vi "sub_conv_map_gen_v2.vi"(11 "code type":T1(ring)) -> (1 "output in decimal":u32[][](array[numeric]), 3 "state transition":u32[][](array[numeric]))   [LabVIEW 2014]
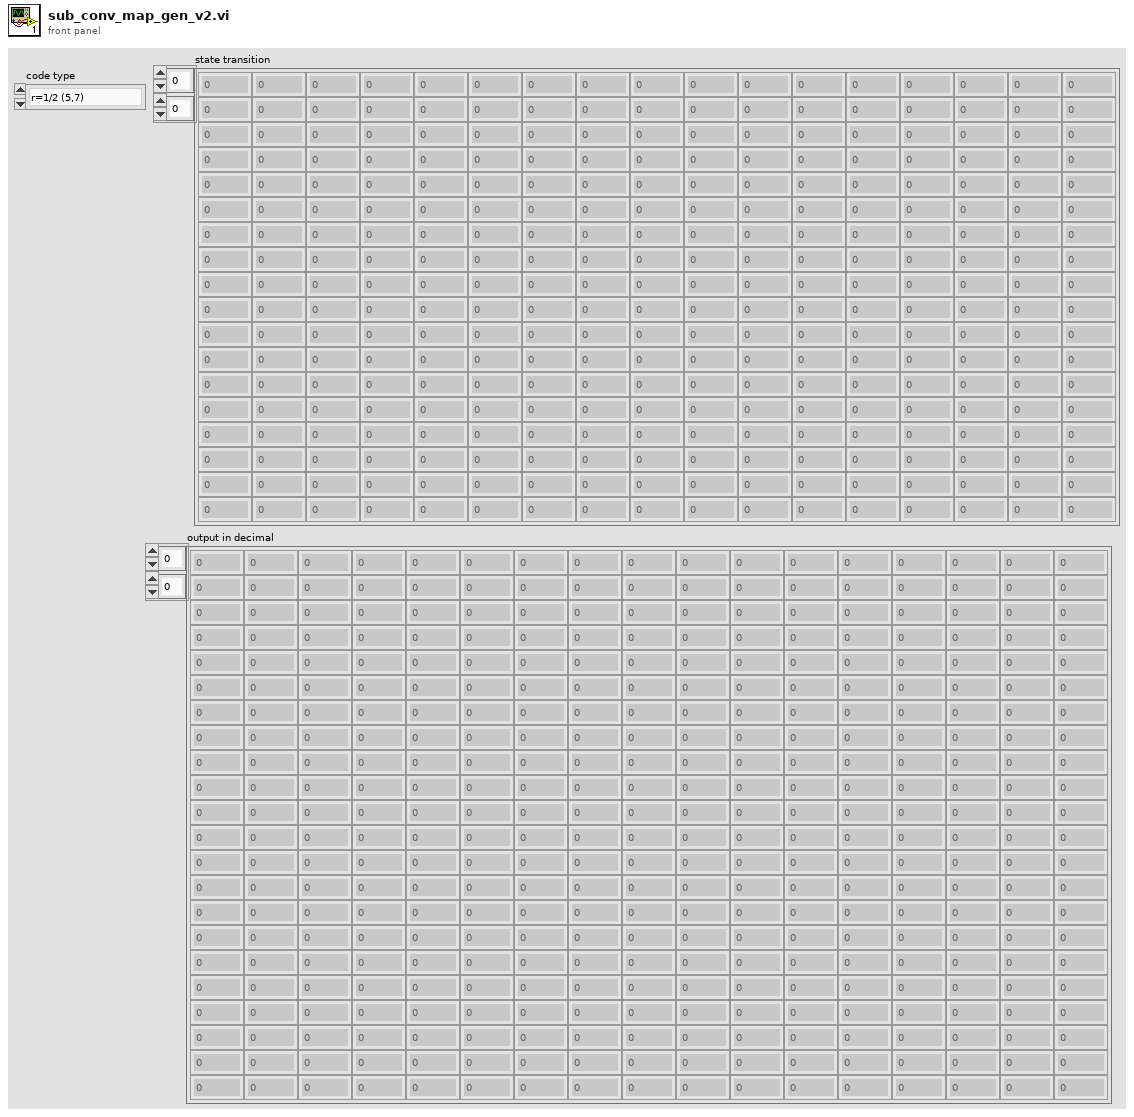
[diagram p1: front panel]
types:
  T1 = enum16{"r=1/2 (5,7)", "r=1/2 (13,17)", "r=1/4 (25,27,33,37)"}
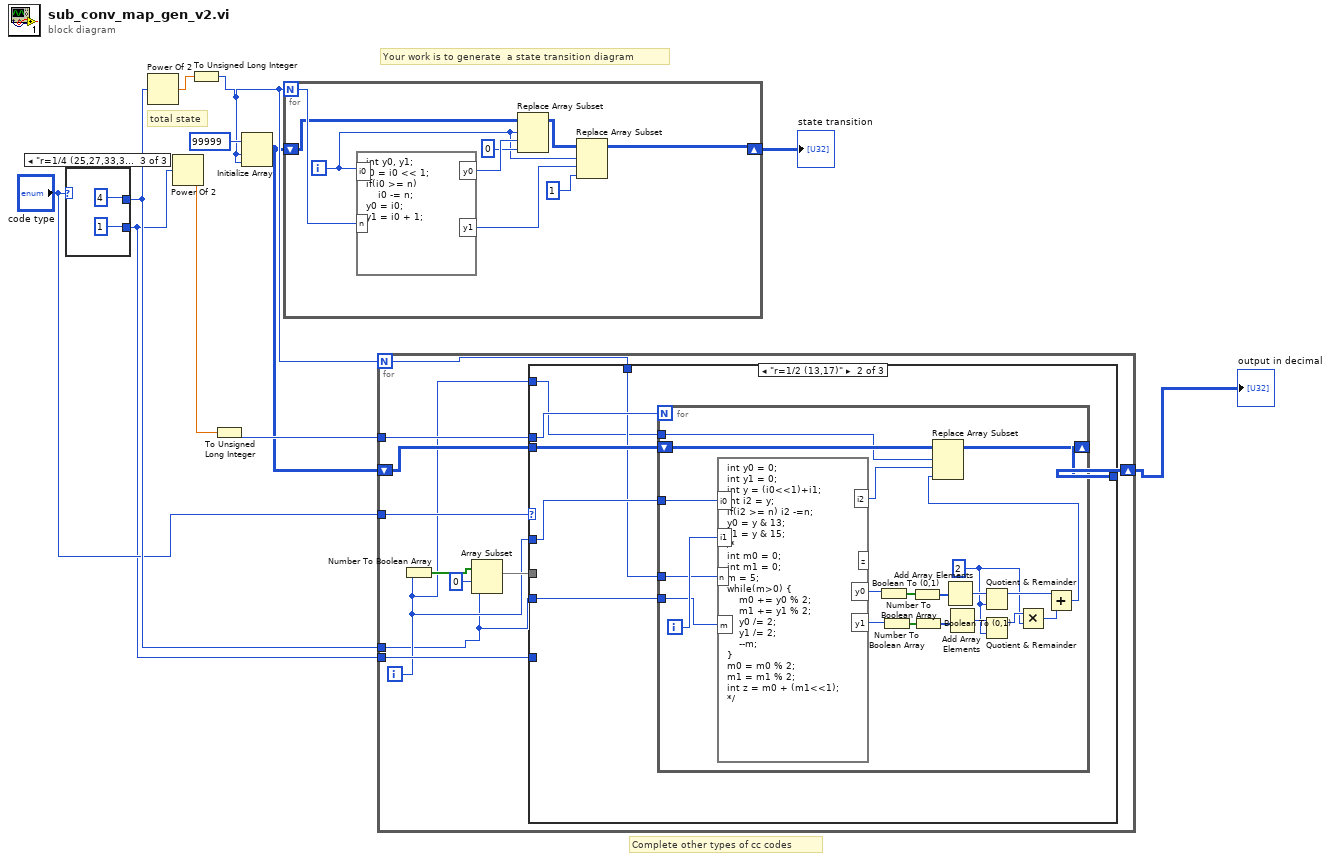
[diagram p0: block diagram]
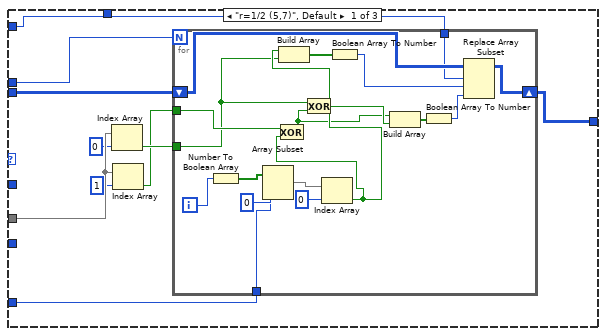
[diagram p2: hidden frame]
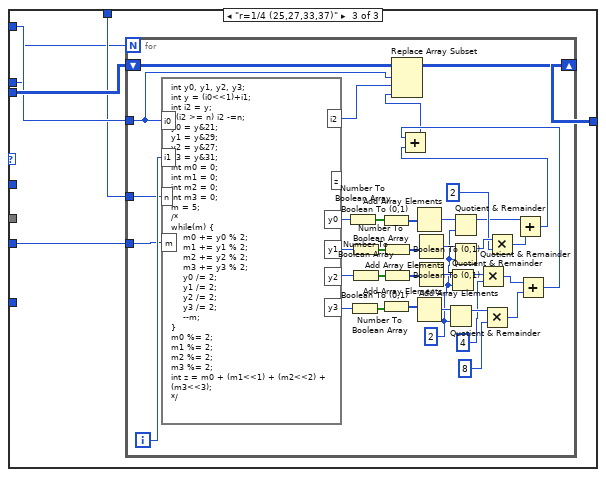
[diagram p3: hidden frame]
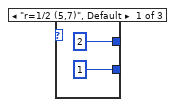
[diagram p4: hidden frame]
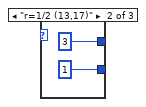
[diagram p5: hidden frame]
diagram:
  # "Your work is to generate  a state transition diagram"
  # "Complete other types of cc codes"
  # "total state"
  n1 = case shown="\"r=1/4 (25,27,33,37)\"" "code type" {
    tunnel: [u32 2 u32 3 u32 4] -> w9
    tunnel: [u32 1 u32 1 u32 1] -> w1
    frame "r=1/2 (5,7)", Default {
    }
    frame "r=1/2 (13,17)" {
    }
    frame "r=1/4 (25,27,33,37)" {
    }
  }
  n2 = Power Of 2(x=w9) -> (2^x=w7:dbl)
  n3 = Power Of 2(x=w1) -> (2^x=w6:dbl)
  n4 = To Unsigned Long Integer(number=w7) -> (unsigned 32bit integer=w4:u32)
  n5 = To Unsigned Long Integer(number=w6) -> (unsigned 32bit integer=w5:u32)
  n6 = Initialize Array(u32 99999, w4, w4) -> (w3:u32[][])
  n7 = for {
    N: w4 -> [w26]
    shift-right: [w18] -> w10
    shift-left: w3 -> [w25]
    i -> [w19]
    n8 = formula code="int y0, y1;\ni0 = i0 << 1;\nif(i0 >= n)\n    i0 -= n;\ny0 = i0;\ny1 = i0 + 1;"("i0"=w19, "n"=w26) -> ("y0"=w23:i32, "y1"=w20:i32)
    n9 = Replace Array Subset(array=w25, new element=0, index (row)=w19, index (col)=w23) -> (w24:u32[][])
    n10 = Replace Array Subset(array=w24, new element=1, index (row)=w19, index (col)=w20) -> (w18:u32[][])
  }
  "state transition" <- w10
  n11 = for {
    N: w4 -> [w28]
    tunnel: w5 -> [w37]
    tunnel: w1 -> [w31]
    tunnel: w9 -> [w27]
    tunnel: "code type" -> [w34]
    shift-right: [w32] -> w2
    shift-left: w3 -> [w33]
    i -> [w29]
    n12 = Number To Boolean Array(number=w29) -> (Boolean array=w36:bool[])
    n13 = Array Subset(array=w36, index=0, length=w27) -> (w35:bool[])
    n14 = case shown="\"r=1/2 (13,17)\"" w34 {
      tunnel: w37 -> [w47 w70 w95]
      tunnel: w31 -> [w46 _ _]
      tunnel: w35 -> [w45 _ _]
      tunnel: [w38 w72 w98] -> w32
      tunnel: w33 -> [w40 w71 w99]
      tunnel: w29 -> [w39 w67 w97]
      tunnel: w29 -> [_ w69 _]
      tunnel: w28 -> [_ w68 w96]
      tunnel: w27 -> [_ w66 w94]
      frame "r=1/2 (5,7)", Default {
        n15 = Index Array(array=w45, index=0) -> (element=w42:bool)
        n16 = Index Array(array=w45, index=1) -> (element=w41:bool)
        n17 = for {
          N: w47 -> [_]
          tunnel: w46 -> [w62]
          tunnel: w41 -> [w51]
          tunnel: w42 -> [w50]
          shift-right: [w53] -> w38
          shift-left: w40 -> [w57]
          tunnel: w39 -> [w55]
          i -> [w65]
          n18 = Number To Boolean Array(number=w65) -> (Boolean array=w64:bool[])
          n19 = Array Subset(array=w64, index=0, length=w62) -> (w61:bool[])
          n20 = Index Array(array=w61, index=0) -> (element=w52:bool)
          n21 = Exclusive Or(1:w52, 2:w51) -> (0:w48:bool)
          n22 = Build Array(w52, w50) -> (w58:bool[])
          n23 = Exclusive Or(1:w48, 2:w50) -> (0:w49:bool)
          n24 = Boolean Array To Number(Boolean array=w58) -> (number=w54:u32)
          n25 = Build Array(w48, w49) -> (w59:bool[])
          n26 = Boolean Array To Number(Boolean array=w59) -> (number=w56:u32)
          n27 = Replace Array Subset(array=w57, new element=w56, index (row)=w55, index (col)=w54) -> (w53:u32[][])
        }
      }
      frame "r=1/2 (13,17)" {
        n28 = for {
          N: w70 -> [_]
          shift-right: [w89] -> w72
          shift-left: w71 -> [w93]
          tunnel: w69 -> [w92]
          tunnel: w68 -> [w90]
          tunnel: w67 -> [w87]
          tunnel: w66 -> [w86]
          i -> [w91]
          w74 = 2
          n29 = formula code="int y0 = 0;\nint y1 = 0;\nint y = (i0<<1)+i1;\nint i2 = y;\nif(i2 >= n) i2 -=n;\ny0 = y & 13;\ny1 = y & 15;\n/*\nint m0 = 0;\nint m1 = 0;\nm = 5;\nwhile(m>0) {\n    m0 += y0 % 2;\n    m1 += y1 % 2;\n    y0 /= 2;\n    y1 /= 2;\n    --m;\n}\nm0 = m0 % 2;\nm1 = m1 % 2;\nint z = m0 + (m1<<1);\n*/"("i0"=w92, "i1"=w91, "n"=w90, "m"=w86) -> ("i2"=w88:i32, "y0"=w76:i32, "y1"=w75:i32)  [unwired: 1 out]
          n30 = Number To Boolean Array(number=w76) -> (Boolean array=w85:bool[])
          n31 = Number To Boolean Array(number=w75) -> (Boolean array=w84:bool[])
          n32 = Boolean To (0,1)(Boolean=w85) -> (0, 1=w82:i16[])
          n33 = Boolean To (0,1)(Boolean=w84) -> (0, 1=w83:i16[])
          n34 = Add Array Elements(numeric array=w82) -> (sum=w81:i16)
          n35 = Add Array Elements(numeric array=w83) -> (sum=w80:i16)
          n36 = Quotient & Remainder(x=w81, y=w74) -> (x-y*floor(x/y)=w77:i32)  [unwired: 1 out]
          n37 = Quotient & Remainder(x=w80, y=w74) -> (x-y*floor(x/y)=w79:i32)  [unwired: 1 out]
          n38 = Multiply(x=w79, y=w74) -> (x*y=w78:i32)
          n39 = Add(x=w77, y=w78) -> (x+y=w73:i32)
          n40 = Replace Array Subset(array=w93, new element=w73, index (row)=w87, index (col)=w88) -> (w89:u32[][])
        }
      }
      frame "r=1/4 (25,27,33,37)" {
        n41 = for {
          N: w95 -> [_]
          shift-right: [w133] -> w98
          shift-left: w99 -> [w136]
          tunnel: w97 -> [w132]
          tunnel: w96 -> [w134]
          tunnel: w94 -> [w130]
          i -> [w135]
          w113 = 2
          n42 = formula code="int y0, y1, y2, y3;\nint y = (i0<<1)+i1;\nint i2 = y;\nif(i2 >= n) i2 -=n;\ny0 = y&21;\ny1 = y&29;\ny2 = y&27;\ny3 = y&31;\nint m0 = 0;\nint m1 = 0;\nint m2 = 0;\nint m3 = 0;\nm = 5;\n/*\nwhile(m) {\n    m0 += y0 % 2;\n    m1 += y1 % 2;\n    m2 += y2 % 2;\n    m3 += y3 % 2;\n    y0 /= 2;\n    y1 /= 2;\n    y2 /= 2;\n    y3 /= 2;\n    --m;\n}\nm0 %= 2;\nm1 %= 2;\nm2 %= 2;\nm3 %= 2;\nint z = m0 + (m1<<1) + (m2<<2) + (m3<<3);\n*/"("i0"=w132, "i1"=w135, "n"=w134, "m"=w130) -> ("i2"=w131:i32, "y0"=w129:i32, "y1"=w128:i32, "y2"=w127:i32, "y3"=w126:i32)  [unwired: 1 out]
          n43 = Number To Boolean Array(number=w129) -> (Boolean array=w125:bool[])
          n44 = Number To Boolean Array(number=w126) -> (Boolean array=w124:bool[])
          n45 = Number To Boolean Array(number=w128) -> (Boolean array=w122:bool[])
          n46 = Number To Boolean Array(number=w127) -> (Boolean array=w123:bool[])
          n47 = Boolean To (0,1)(Boolean=w125) -> (0, 1=w118:i16[])
          n48 = Boolean To (0,1)(Boolean=w124) -> (0, 1=w121:i16[])
          n49 = Boolean To (0,1)(Boolean=w122) -> (0, 1=w119:i16[])
          n50 = Boolean To (0,1)(Boolean=w123) -> (0, 1=w120:i16[])
          n51 = Add Array Elements(numeric array=w118) -> (sum=w117:i16)
          n52 = Add Array Elements(numeric array=w121) -> (sum=w116:i16)
          n53 = Add Array Elements(numeric array=w119) -> (sum=w114:i16)
          n54 = Add Array Elements(numeric array=w120) -> (sum=w115:i16)
          n55 = Quotient & Remainder(x=w116, y=w113) -> (x-y*floor(x/y)=w112:i32)  [unwired: 1 out]
          n56 = Quotient & Remainder(x=w115, y=w113) -> (x-y*floor(x/y)=w111:i32)  [unwired: 1 out]
          n57 = Quotient & Remainder(x=w117, y=w113) -> (x-y*floor(x/y)=w105:i32)  [unwired: 1 out]
          n58 = Quotient & Remainder(x=w114, y=w113) -> (x-y*floor(x/y)=w108:i32)  [unwired: 1 out]
          n59 = Multiply(x=w111, y=4) -> (x*y=w104:i32)
          n60 = Multiply(x=w112, y=8) -> (x*y=w103:i32)
          n61 = Multiply(x=w108, y=2) -> (x*y=w106:i32)
          n62 = Add(x=w105, y=w106) -> (x+y=w102:i32)
          n63 = Add(x=w104, y=w103) -> (x+y=w101:i32)
          n64 = Add(x=w101, y=w102) -> (x+y=w100:i32)
          n65 = Replace Array Subset(array=w136, new element=w100, index (row)=w132, index (col)=w131) -> (w133:u32[][])
        }
      }
    }
  }
  "output in decimal" <- w2
